vi "Ramsete_Diff_DO_SI.vi"(5 "WheelBase-Meters":dbl=2.0, 6 "Gyro-Radians":dbl, 7 "Reset":bool, 8 "RightDist-Meters":dbl, 9 "LeftDist-Meters":dbl, 10 "TRAJ_STATE":T5={"TimeSeconds"=0.0, "Velocity"=0.0, "Acceleration"=0.0, "POSE"={"TRANSLATION"={"X"=0.0, "Y"=0.0}, "ROTATION"={"VALUE"=0.0, "COS"=1.0, "SIN"=0.0}}, "Curvature"=0.0} {"POSE"."ROTATION"."SIN" format="%13.4f"; "POSE"."ROTATION"."COS" format="%13.4f"; "POSE"."ROTATION"."VALUE" format="%13.4f"; "POSE"."TRANSLATION"."Y" format="%14.3f"; "POSE"."TRANSLATION"."X" format="%14.3f"}, 11 "inRAMSETE":T1={"B"=2.0, "Zeta"=0.7, "poseTolerance"={"TRANSLATION"={"X"=0.0, "Y"=0.0}, "ROTATION"={"VALUE"=0.0, "COS"=1.0, "SIN"=0.0}}, "poseError"={"TRANSLATION"={"X"=0.0, "Y"=0.0}, "ROTATION"={"VALUE"=0.0, "COS"=1.0, "SIN"=0.0}}, "Enabled"=TRUE} {"poseError"."ROTATION"."SIN" format="%13.4f"; "poseError"."ROTATION"."COS" format="%13.4f"; "poseError"."ROTATION"."VALUE" format="%13.4f"; "poseError"."TRANSLATION"."Y" format="%14.3f"; "poseError"."TRANSLATION"."X" format="%14.3f"; "poseTolerance"."ROTATION"."SIN" format="%13.4f"; "poseTolerance"."ROTATION"."COS" format="%13.4f"; "poseTolerance"."ROTATION"."VALUE" format="%13.4f"; "poseTolerance"."TRANSLATION"."Y" format="%14.3f"; "poseTolerance"."TRANSLATION"."X" format="%14.3f"; "Zeta" format="%12.3f"; "B" format="%12.3f"}) -> (0 "AtReference":bool, 1 "RightVelDmd":dbl, 2 "LeftVelDmd":dbl, 3 "outRAMSETE":T1={"B"=2.0, "Zeta"=0.7, "poseTolerance"={"TRANSLATION"={"X"=0.0, "Y"=0.0}, "ROTATION"={"VALUE"=0.0, "COS"=1.0, "SIN"=0.0}}, "poseError"={"TRANSLATION"={"X"=0.0, "Y"=0.0}, "ROTATION"={"VALUE"=0.0, "COS"=1.0, "SIN"=0.0}}, "Enabled"=TRUE} {"poseError"."ROTATION"."SIN" format="%13.4f"; "poseError"."ROTATION"."COS" format="%13.4f"; "poseError"."ROTATION"."VALUE" format="%13.4f"; "poseError"."TRANSLATION"."Y" format="%14.3f"; "poseError"."TRANSLATION"."X" format="%14.3f"; "poseTolerance"."ROTATION"."SIN" format="%13.4f"; "poseTolerance"."ROTATION"."COS" format="%13.4f"; "poseTolerance"."ROTATION"."VALUE" format="%13.4f"; "poseTolerance"."TRANSLATION"."Y" format="%14.3f"; "poseTolerance"."TRANSLATION"."X" format="%14.3f"; "Zeta" format="%12.3f"; "B" format="%12.3f"}, 4 "CurrentRelativePose":T2 {"ROTATION"."SIN" format="%13.4f"; "ROTATION"."COS" format="%13.4f"; "ROTATION"."VALUE" format="%13.4f"; "TRANSLATION"."Y" format="%14.3f"; "TRANSLATION"."X" format="%14.3f"})   [LabVIEW 2019]
doc: "This is a convience function that takes sensor data, and trajectory demands, then performs differential drive odometry, and executes ramsete control to output wheel speed demands.\n\nAll input and output units are Meters, Radians.\n\nParameters:\n - InRamsete - Ramsete data structure\n - LeftDist - Left wheel distance\n - RightDist - Right wheel distance\n - Gyro - Robot gyro reading\n - Reset - Reset's the internal saved robot position, left / right distance, and gyro readings. This should be set true at the beginning of executing a trajectory.\n - TrajState - The desired trajectory state\n - WheelBase - The robot wheel base\n\nReturns:\n - outRamsete - Updated Ramsete data structure\n - AtReference - TRUE when robot position is withing tolerance\n - CurrentPose - Current robot Pose\n - LeftVelDmd - Left wheel velocity demand (These demands are NOT normalized.)\n -RightVelDmd - Right wheel velocity demand (These demands are NOT normalized.)"
uses:
  TypeDef/POSE2D.ctl
  TypeDef/TRANSLATION2D.ctl
  TypeDef/ROTATION2D.ctl
  TypeDef/TRAJ_STATE.ctl
  TypeDef/RAMSETE.ctl
  <vilib>/Rock Robotics/SystemInterfaces/NetworkCommunication/NetComm_UsageReport_report.vi
  Globals/Util_LibraryGlobals.vi
  Trajectory_Library.lvlib
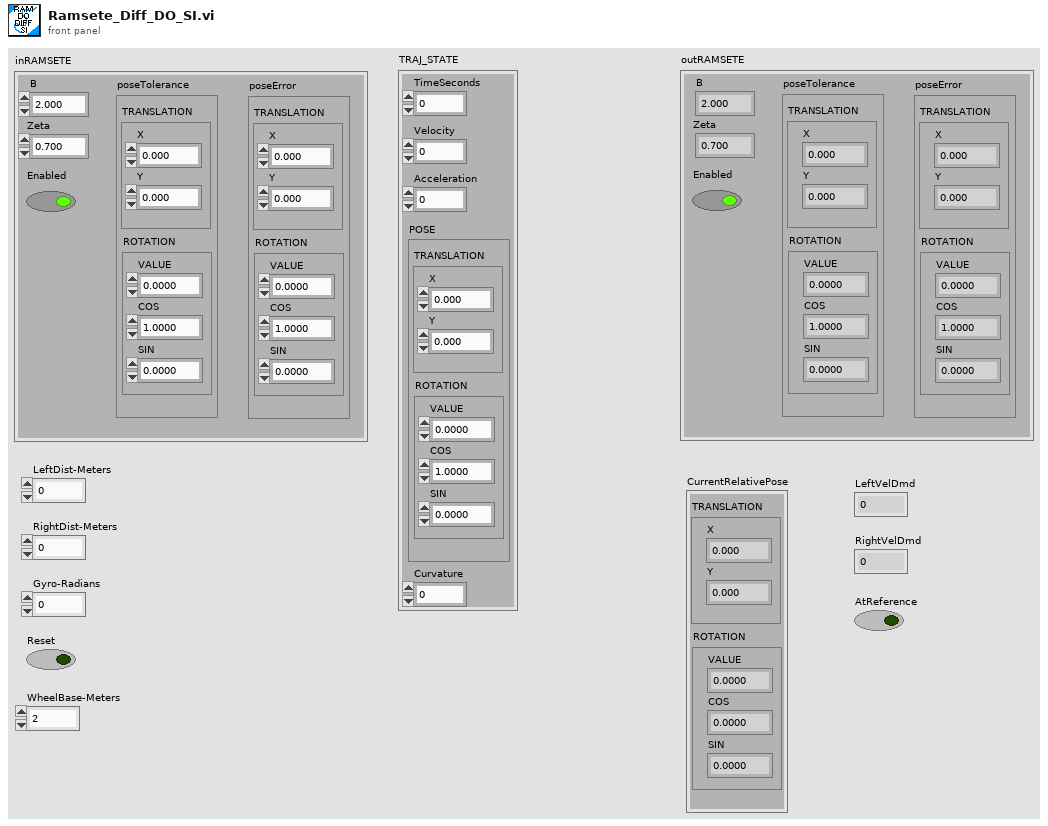
[diagram p1: front panel]
types:
  T1 = typedef "Trajectory_Library.lvlib/RAMSETE.ctl" = cluster{"B":dbl, "Zeta":dbl, "poseTolerance":T2, "poseError":T2, "Enabled":bool}
  T2 = typedef "Trajectory_Library.lvlib/POSE2D.ctl" = cluster{"TRANSLATION":T3, "ROTATION":T4}
  T3 = typedef "Trajectory_Library.lvlib/TRANSLATION2D.ctl" = cluster{"X":dbl, "Y":dbl}
  T4 = typedef "Trajectory_Library.lvlib/ROTATION2D.ctl" = cluster{"VALUE":dbl, "COS":dbl, "SIN":dbl}
  T5 = typedef "Trajectory_Library.lvlib/TRAJ_STATE.ctl" = cluster{"TimeSeconds":dbl, "Velocity":dbl, "Acceleration":dbl, "POSE":T2, "Curvature":dbl}
  T6 = typedef "Trajectory_Library.lvlib/DIFF_DRIVE_KINEMATICS.ctl" = cluster{"TrackWidth_Meters":dbl}
  T7 = typedef "Trajectory_Library.lvlib/CHASSIS_SPEEDS.ctl" = cluster{"vX":dbl, "vY":dbl, "vOmega":dbl}
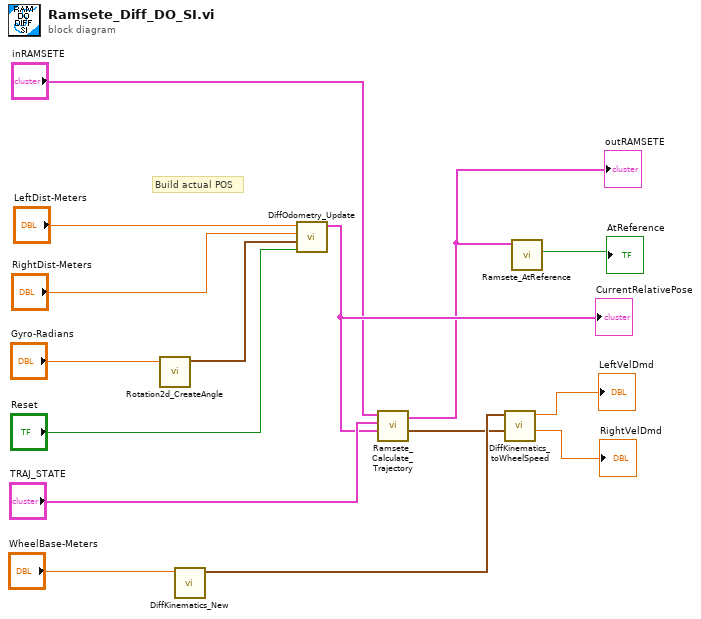
[diagram p0: block diagram]
diagram:
  # "Build actual POS"
  n1 = call "Rotation2d_CreateAngle.vi"("Angle"="Gyro-Radians") -> ("ROTATION"=w10:T4)  [unwired: 10 in]
  n2 = call "DiffKinematics_New.vi"("TrackWidth_Meters"="WheelBase-Meters") -> ("DIFF_DRIVE_KINEMATICS"=w8:T6)  [unwired: 10 in]
  n3 = call "DiffOdometry_Update.vi"("Reset"="Reset", "Heading"=w10, "RightDistance"="RightDist-Meters", "LeftDistance"="LeftDist-Meters") -> ("CurrentRelativePose"=w4:T2)  [unwired: 7 in]
  "CurrentRelativePose" <- w4
  n4 = call "Ramsete_Calculate_Trajectory.vi"("CurrentPOSE"=w4, "TRAJ_STATE"="TRAJ_STATE", "inRAMSETE"="inRAMSETE") -> ("CHASSIS Speeds"=w6:T7, "outRAMSETE"=w3:T1)  [unwired: 7 in]
  "outRAMSETE" <- w3
  n5 = call "DiffKinematics_toWheelSpeed.vi"("CHASSIS Speed"=w6, "DIFF_DRIVE_KINEMATICS"=w8) -> ("RightVelocity"=→"RightVelDmd":dbl, "LeftVelocity"=→"LeftVelDmd":dbl)  [unwired: 8 in]
  n6 = call "Ramsete_AtReference.vi"("RAMSETE"=w3) -> ("AtReference"=→"AtReference":bool)  [unwired: 10 in]
